vi "FGPA Area FWHM.vi"() -> ()   [LabVIEW 2017]
uses:
  <vilib>/rvi/interface/nirviOpenFPGA/nirviOpenFPGA.xnode
  <vilib>/rvi/interface/nirviCloseFPGA/nirviCloseFPGA.xnode
  <vilib>/rvi/Analysis/host/Public/NI_FpgaMspHost.lvlib
  <vilib>/rvi/interface/nirviMethod/nirviMethod.xnode
  <vilib>/rvi/errors/niLvFpgaMergeErrorWithErrorCode.vi
  <vilib>/FPGAPlugInAG/Dynamic/niLvFpga_Run_Dynamic.vi
  <vilib>/FPGAPlugInAG/Dynamic/niLvFpga_Reset_Dynamic.vi
  <vilib>/FPGAPlugInAG/Dynamic/niLvFpga_ConfigureFifo_Dynamic.vi
  <vilib>/FPGAPlugInAG/Dynamic/niLvFpga_ReadFifo_Dynamic.vi
  <vilib>/rvi/interface/nirviReadWriteControl/nirviReadWriteControl.xnode
  <extravilib>/ChannelInstances/Tag-bool.lvlib
  <vilib>/Analysis/NI_AALBase.lvlib
  FPGA Bitfiles/FPGAAreaFWHM_FPGATarget_ReadAnalog3Pulse_FqF0E97EYxI.lvbitx
  FADS_Area FWHM.vi
  <vilib>/Analysis/baseanly.llb/Mean (DBL).vi
  <vilib>/Utility/file.llb/Write Delimited Spreadsheet (DBL).vi
  <vilib>/rvi/Analysis/host/Private/Sample Rate To Loop Time (ticks).vi
  <vilib>/rvi/interface/Simulation/niFpgaSimulationCallBeginRW.vi
  <vilib>/rvi/errors/niLvFpgaAdjustHostInterfaceError.vi
  <vilib>/FPGAPlugInAG/Dynamic/niLvFpga_Close_Dynamic.vi
panel:
  out "Droplet Rate":dbl format="%0.2f"
  in  "Sample Name":string
  in  "Folder For Plots":path
  in  "Log Sorted Drop Data":bool
  in  "Tab Control":enum32{"Width", "FWHM"}(tab)
  in  "Min Width (us)":u32
  in  "Max Width (us)":u32=10000
  in  "Min FWHM (us)":i32
  in  "Max FWHM (us)":i32=10000
  out "Combined Histogram":T1(graph)
  out "Outside Sorted":cluster{"total":i32, "below":i32, "above":i32}
  out "Histogram Sorted Drops":T2(graph)
  out "Voltage Bins":i32
  out "Histogram":T2(graph)
  out "Outside Unsorted":cluster{"total":i32, "below":i32, "above":i32}
  out "Fraction Sorted":dbl
  out "Total Number of Droplets":i32
  out "Area Amplitude":i32[][](graph) caption="Area vs Amplitude"
  out "Area Bin Size":i32
  out "Voltage Bin Size":dbl=0.005
  in  "stop":bool
  out "FWHM Amplitude":i32[][](graph) caption="FWHM vs Amplitude"
  out "Buffer":u32
  out "Loop Time (ms)":u32
  out "Data Transfer":bool
  in  "Sort":bool
  out "Width Bin Size":i32
  in  "Save Plots":bool caption="Enable"
  out "Width Amplitude":i32[][](graph) caption="Width vs Amplitude"
  in  "Max Voltage (V)":dbl=10.0
  in  "Min Voltage (V)":dbl=10.0
  in  "Noise Level":dbl=0.2
  out "Sorted Droplets":u32
  in  "PMT Voltage":dbl(slide) scale=0.0..1.25
  in  "Add":bool
  in  "Reset":bool
  out "Voltage Trace":cluster{dbl[], dbl[]}[](graph)
  out "Sample Rate":dbl format="%#_6p"
  # "SORTING SETTINGS"
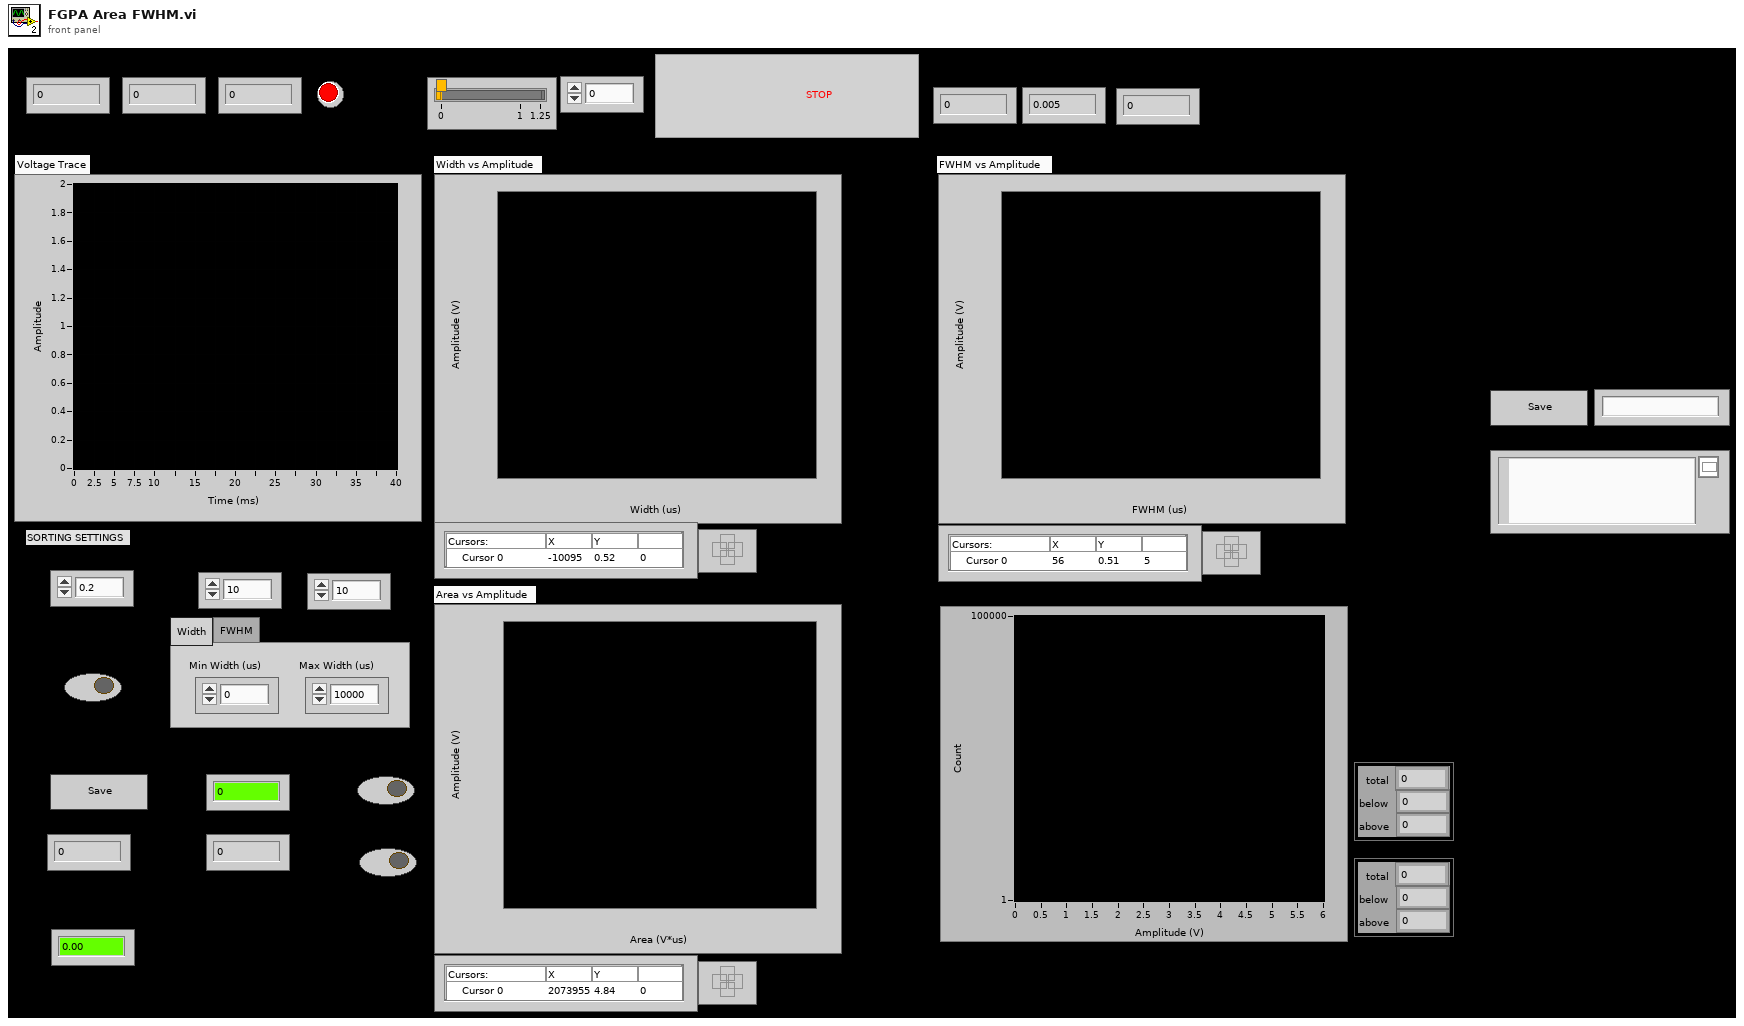
[diagram p1: front panel]
types:
  T1 = cluster{"X Values":dbl[], "Histogram: h(x)":i32[]}[]
  T2 = cluster{"X Values":dbl[], "Histogram: h(x)":i32[]}
  T3 = typedef "Tag-bool.lvlib/))Channel.ctl" = refnum<queue>
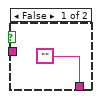
[diagram p3: hidden frame]
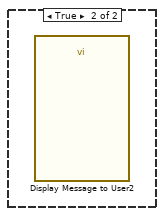
[diagram p4: hidden frame]
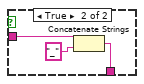
[diagram p6: hidden frame]
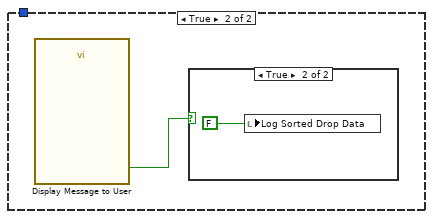
[diagram p7: hidden frame]
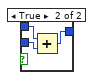
[diagram p9: hidden frame]
diagram:
  n1 = flat-sequence {
    tunnel: [w13] -> w5
    tunnel: [w12] -> w4
    tunnel: [w11] -> w3
    tunnel: [w10] -> w2
    tunnel: [w9] -> w1
    tunnel: [w47] -> w8
    tunnel: [w46] -> w7
    tunnel: [w45] -> w6
    tunnel: w5 -> [w44]
    tunnel: w4 -> [w43]
    tunnel: w3 -> [w42]
    tunnel: w2 -> [w39]
    tunnel: w1 -> [w41]
    tunnel: w8 -> [w317]
    tunnel: w7 -> [w316]
    tunnel: w6 -> [w315]
    frame #0 {
      w36 = 1000.0 ("x")
      w24 = 0.005 ("Voltage Bin Size")
      w11 = u32 100 ("milliseconds to wait")
      w32 = 0 ("element")
      # "Area Bin"
      # "INITIALIZE ARRAY WITH CORRECT BINS"
      # "Max Width Size"
      n2 = call-poly <vilib>:"Sample Rate To Loop Time.vi"("sample rate (S/s)"=200000.0 ("FPGA clock rate (Hz)"), "FPGA clock rate (Hz)"=40000000.0) -> ("actual sample rate (S/s)"=w38:dbl)  [unwired: 11 in, 2 out]
      "Sample Rate" <- w38
      n3 = Reciprocal(x=w38) -> (1/x=w9:dbl)
      n4 = Reciprocal(x=w38) -> (1/x=w20:dbl)
      n5 = Multiply(x=1000000.0, y=w20) -> (x*y=w19:dbl)
      n6 = Multiply(x=2.0, y=w19) -> (x*y=w14:dbl)
      n7 = To Long Integer(number=w14) -> (32bit integer=→"Width Bin Size":i32)
      n8 = Divide(x=10000.0 ("Max Width"), y=w14) -> (x/y=w22:dbl)
      n9 = Divide(x=11.0, y=w24) -> (x/y=w21:dbl)
      n10 = Divide(x=w38, y=1000.0) -> (x/y=w27:dbl)
      n11 = To Long Integer(number=w21) -> (32bit integer=w31:i32)
      "Voltage Bins" <- w31
      n12 = To Long Integer(number=w22) -> (32bit integer=w16:i32)
      n13 = Multiply(x=w11, y=w27) -> (x*y=w29:dbl)
      n14 = Initialize Array(w32, w16, w31) -> (w12:i32[][])
      n15 = To Unsigned Long Integer(number=w29) -> (unsigned 32bit integer=w10:u32)
      n16 = Divide(x=5000000.0, y=w36) -> (x/y=w35:dbl)
      n17 = To Long Integer(number=w35) -> (32bit integer=w34:i32)
      n18 = To Long Integer(number=w36) -> (32bit integer=→"Area Bin Size":i32)
      n19 = Initialize Array(w32, w34, w31) -> (w13:i32[][])
      "Voltage Bin Size" <- w24
    }
    frame #1 {
      w49 = u32 40000 ("Requested Depth")
      n20 = xnode "Open FPGA VI Reference"() -> ("FPGA VI Reference Out"=w69:refnum<k20>, "error out"=w65:errorcluster)  [unwired: 2 in]
      n21 = xnode "Invoke Method"("FPGA VI Reference In"=w69, "error in"=w65) -> ("FPGA VI Reference Out"=w66:refnum<k20>, "error out"=w64:errorcluster)
      n22 = xnode "Invoke Method"("FPGA VI Reference In"=w66, "error in"=w64, "Requested Depth"=w49) -> ("FPGA VI Reference Out"=w68:refnum<k20>, "error out"=w67:errorcluster)  [unwired: 1 out]
      n23 = xnode "Invoke Method"("FPGA VI Reference In"=w68, "Requested Depth"=w49) -> ("FPGA VI Reference Out"=w59:refnum<k20>)  [unwired: 1 in, 2 out]
      n24 = xnode "Invoke Method"("FPGA VI Reference In"=w59, "Requested Depth"=w49) -> ("FPGA VI Reference Out"=w50:refnum<k20>)  [unwired: 1 in, 2 out]
      n25 = xnode "Invoke Method"("FPGA VI Reference In"=w50, "error in"=w67) -> ("FPGA VI Reference Out"=w56:refnum<k20>, "error out"=w54:errorcluster)  [unwired: 1 in]
      n26 = Initialize Array(0.0 ("element"), 20 ("dimension size")) -> (w62:dbl[])
      n27 = for {
        N: w39 -> [_]
        tunnel: [w88] -> w57 mode=indexing
        tunnel: w41 -> [w87]
        i -> [w90]
        n28 = To Double Precision Float(number=w90) -> (double precision float=w89:dbl)
        n29 = Multiply(x=w87, y=w89) -> (x*y=w88:dbl)
      }
      n30 = Multiply(x=u32 2, y=w39) -> (x*y=w40:u32)
      n31 = Multiply(x=1000.0, y=w57) -> (x*y=w55:dbl[])
      n32 = while {
        tunnel: w56 -> [w86]
        tunnel: w55 -> [w72]
        tunnel: w42 -> [w82]
        tunnel: w40 -> [w84]
        tunnel: w54 -> [w81]
        tunnel: [w80] -> w45
        tunnel: [w76] -> w53
        stop <- w77 stop-if-true
        # "Data Stean of Voltage Trace"
        n33 = Wait (ms)(milliseconds to wait=w82) -> ()  [unwired: 1 out]
        n34 = xnode "Invoke Method"("FPGA VI Reference In"=w86, "error in"=w81, "Number of Elements"=w84, "Timeout (ms)"=5000) -> ("error out"=w80:errorcluster, "Data"=w85:void[])  [unwired: 2 out]
        n35 = call "Conversion_to_Volt.vi"("Data"=w85) -> ("Array"=w71:dbl[])  [unwired: 10 in]
        n36 = Decimate 1D Array(w71) -> (w75:dbl[], w73:dbl[])
        n37 = Bundle(w72, w75) -> ()  [unwired: 1 in, 1 out]
        n38 = Bundle(w72, w73) -> (w70:cluster{dbl[], dbl[]})  [unwired: 1 in]
        n39 = Build Array(w70) -> (→"Voltage Trace":cluster{dbl[], dbl[]}[])
        n40 = Unbundle By Name(w80) -> ("status"=w79:bool)
        n41 = Or(x=w79, y="stop") -> (x .or. y?=w77:bool)
        n42 = call <extravilib>:"Write.vi"("element"=w77) -> ("channel"=w76:T3)  [unwired: 1 out]
      }
      n43 = while {
        shift-right: [w200] -> w46
        shift-left: w54 -> [w225]
        shift-right: [w156] -> w47
        shift-left: w56 -> [w228]
        shift-right: [w220] -> _
        shift-left: w62 -> [w221]
        shift-right: [w213] -> _
        shift-left: 0 ("dimension size") -> [w214]
        shift-right: [w178] -> _
        shift-left: u32 0 ("millisecond timer value") -> [w179]
        tunnel: w43 -> [w170]
        tunnel: w53 -> [w162]
        tunnel: w44 -> [w148]
        shift-right: [w135] -> _
        shift-left: 0 -> [w138]
        stop <- w224 stop-if-true
        w116 = 0.0 ("min")
        w115 = 11.0 ("max")
        w150 = u32 4
        w175 = u32 4 ("y")
        # "Collected Drops"
        # "To Waste Drops"
        # "All Drops"
        # "PLOT FILTERED CUMULATED 1D HISTOGRAM OF PEAK AMPLITUDE"
        # "Area"
        # "FWHM"
        # "Width"
        # "FWHM"
        # "Area"
        # "Amplitude"
        # "Width"
        # "Check for Data Transfer Slippage"
        # "Amplitude"
        # "NUMBER OF SAMPLES MULTIPLE OF FOUR"
        # "Write to FPGA Controls and Read from FPGA Indicators"
        n44 = local read "Reset"() -> (w192:bool)
        n45 = Wait (ms)(milliseconds to wait=u32 100) -> ()  [unwired: 1 out]
        n46 = call "Conversion.vi"("Sorting Threshold"="Max Voltage (V)") -> ("Numeric 2"=w189:i16)  [unwired: 9 in, 1 out]
        n47 = call "Conversion.vi"("Sorting Threshold"="Noise Level") -> ("Numeric 2"=w206:i16)  [unwired: 9 in, 1 out]
        n48 = call "Conversion.vi"("Sorting Threshold"="PMT Voltage") -> ("Numeric 2"=w212:i16)  [unwired: 9 in, 1 out]
        n49 = call "Conversion.vi"("Sorting Threshold"="Min Voltage (V)") -> ("Numeric 2"=w188:i16)  [unwired: 9 in, 1 out]
        n50 = Equal?(x="Tab Control", y=enum32{"Width", "FWHM"}."FWHM") -> (x = y?=w104:bool)
        n51 = Tick Count (ms)() -> (millisecond timer value=w178:u32)
        n52 = Equal?(x=20, y=w214) -> (x = y?=w216:bool)
        n53 = Subtract(x=w178, y=w179) -> (x-y=→"Loop Time (ms)":u32)
        n54 = xnode "Read/Write Control"("FPGA VI Reference In"=w228, "error in"=w225, "PMT Voltage"=w212, "Noise Level"=w206, "Min Sorting Threshold"=w188, "Max Sorting Threshold"=w189, "Min Width"="Min Width (us)", "Max Width"="Max Width (us)", "Count Reset"=w192, "Sort"="Sort", "Trigger Length"=u32 50, "Min FWHM"="Min FWHM (us)", "Max FWHM"="Max FWHM (us)", "FWHM"=w104) -> ("FPGA VI Reference Out"=w227:refnum<k20>, "error out"=w226:errorcluster, "Event Count"=→"Sorted Droplets")
        n55 = Increment(x=w214) -> (x+1=w215:i32)
        n56 = Select(t=0, s=w216, f=w215) -> (s? t:f=w213:i32)
        n57 = xnode "Invoke Method"("FPGA VI Reference In"=w227, "error in"=w226, "Number of Elements"=u32 0, "Timeout (ms)"=-1) -> ("FPGA VI Reference Out"=w210:refnum<k20>, "error out"=w201:errorcluster, "Elements Remaining"=w176)  [unwired: 1 out]
        "Buffer" <- w176
        n58 = Quotient & Remainder(x=w176, y=w175) -> (floor(x/y)=w174:u32)  [unwired: 1 out]
        n59 = Multiply(x=w174, y=w175) -> (x*y=w173:u32)
        n60 = xnode "Invoke Method"("FPGA VI Reference In"=w210, "error in"=w201, "Number of Elements"=w173, "Timeout (ms)"=-1) -> ("FPGA VI Reference Out"=w184:refnum<k20>, "error out"=w200:errorcluster, "Data"=w125:void[])  [unwired: 1 out]
        n61 = xnode "Invoke Method"("FPGA VI Reference In"=w184, "Number of Elements"=u32 0, "Timeout (ms)"=-1) -> ("FPGA VI Reference Out"=w157:refnum<k20>, "Elements Remaining"=w152)  [unwired: 1 in, 2 out]
        n62 = Quotient & Remainder(x=w152, y=w150) -> (floor(x/y)=w149:u32)  [unwired: 1 out]
        n63 = Multiply(x=w149, y=w150) -> (x*y=w151:u32)
        n64 = local read "Folder For Plots"() -> (w91:path)
        n65 = xnode "Invoke Method"("FPGA VI Reference In"=w157, "Number of Elements"=w151, "Timeout (ms)"=-1) -> ("FPGA VI Reference Out"=w156:refnum<k20>, "Data"=w124:void[])  [unwired: 1 in, 2 out]
        n66 = local read "Add"() -> (w95:bool)
        n67 = And(x=w95, y="Log Sorted Drop Data") -> (x .and. y?=w94:bool)
        n68 = Insert Into Array(array=w124, new element=w125) -> (w141:void[])  [unwired: 1 in]
        n69 = Decimate 1D Array(w125) -> (w121:void[])  [unwired: 3 out]
        n70 = Decimate 1D Array(w124) -> (w101:void[], w122:void[], w99:void[], w100:void[])
        n71 = Decimate 1D Array(w141) -> (w140:void[], w185:void[], w108:void[], w168:void[])
        n72 = To Word Integer(number=w121) -> (16bit integer=w126:i16[])
        n73 = local read "Loop Time (ms)"() -> (w197:u32)
        n74 = To Word Integer(number=w122) -> (16bit integer=w123:i16[])
        n75 = Absolute Value(x=w108) -> (abs(x)=w107:dbl[])
        n76 = call "Conversion_to_Volt.vi"("Data"=w126) -> ("Array"=w120:dbl[])  [unwired: 10 in]
        n77 = call "Conversion_to_Volt.vi"("Data"=w123) -> ("Array"=w102:dbl[])  [unwired: 10 in]
        n78 = case shown="True" w94 {
          tunnel: w102 -> [_ w290]
          tunnel: w101 -> [_ w289]
          tunnel: w100 -> [_ w288]
          tunnel: w99 -> [_ w287]
          tunnel: w91 -> [_ w283]
          frame False {
          }
          frame True {
            n79 = Multiply(x=w289, y=-1) -> (x*y=w286:i32)
            n80 = Absolute Value(x=w287) -> (abs(x)=w284:dbl[])
            n81 = Equal?(x=w283, y=path "") -> (x = y?=w281:bool)
            n82 = case shown="False" w281 {
              tunnel: w290 -> [w304 _]
              tunnel: w288 -> [w303 _]
              tunnel: w286 -> [w302 _]
              tunnel: w284 -> [w301 _]
              tunnel: w283 -> [w293 _]
              frame False {
                w299 = TRUE ("append to file? (new file:F)")
                n83 = local read "Sample Name"() -> (w291:string)
                n84 = Build Array(w302, w303, w301, w304) -> (w300:dbl[])
                n85 = Not Equal?(x="", y=w291) -> (x != y?=w296:bool)
                n86 = case shown="False" w296 {
                  tunnel: w291 -> [_ w307]
                  tunnel: ["Sample" ("WidthVsAmplitude") w306] -> w294
                  frame False {
                  }
                  frame True {
                    n87 = Concatenate Strings(w307, "_") -> (w306:string)
                  }
                }
                n88 = Concatenate Strings(w294, "SortedDropProperties.txt" ("WidthVsAmplitude")) -> (w297:string)
                n89 = Build Path(base path=w293, name or relative path=w297) -> (appended path=w292:path)
                n90 = call-poly <vilib>:"Write Delimited Spreadsheet.vi"("file path (dialog if empty)"=w292, "2D data"=w300, "append to file? (new file:F)"=w299, "transpose? (no:F)"=w299) -> ()  [unwired: 10 in, 2 out]
              }
              frame True {
                n91 = call "Display Message to User"() -> ("OK"=w309:bool)  [unwired: 10 in, 1 out]
                n92 = case shown="True" w309 {
                  frame False {
                  }
                  frame True {
                    n93 = local write "Log Sorted Drop Data"(FALSE) -> ()
                  }
                }
              }
            }
          }
        }
        n94 = Greater?(x=0 ("y"), y=w140) -> (0:w181:bool)
        n95 = To Double Precision Float(number=w197) -> (double precision float=w198:dbl)
        n96 = Multiply(x=w140, y=-1) -> (x*y=w165:i32)
        n97 = Divide(x=w198, y=1000.0) -> (x/y=w196:dbl)
        n98 = And Array Elements(Boolean array=w181) -> (logical AND=→"Data Transfer":bool)
        n99 = Array Size(array=w140) -> (size(s)=w131:i32)
        n100 = To Double Precision Float(number=w131) -> (double precision float=w195:dbl)
        n101 = Divide(x=w195, y=w196) -> (x/y=w222:dbl)
        n102 = Replace Array Subset(array=w221, new element=w222, index=w214) -> (w220:dbl[])
        n103 = local read "Add"() -> (w132:bool)
        n104 = call-poly <vilib>:"Mean.vi"("X"=w220) -> ("mean"=→"Droplet Rate":dbl)  [unwired: 1 out]
        n105 = case shown="False" w132 {
          tunnel: w138 -> [w311 w314]
          tunnel: w131 -> [_ w313]
          tunnel: [w311 w312] -> w134
          frame False {
          }
          frame True {
            n106 = Add(x=w314, y=w313) -> (x+y=w312:i32)
          }
        }
        "Total Number of Droplets" <- w134
        n107 = local read "Sorted Droplets"() -> (w137:u32)
        n108 = local read "Reset"() -> (w133:bool)
        n109 = To Word Integer(number=w185) -> (16bit integer=w186:i16[])
        n110 = call "Conversion_to_Volt.vi"("Data"=w186) -> ("Array"=w127:dbl[])  [unwired: 10 in]
        n111 = Divide(x=w137, y=w134) -> (x/y=→"Fraction Sorted":dbl)
        n112 = local read "Voltage Bin Size"() -> (w142:dbl)
        n113 = local read "Width Bin Size"() -> (w166:i32)
        n114 = local read "Width Bin Size"() -> (w169:i32)
        n115 = Select(t=w131, s=w133, f=w134) -> (s? t:f=w135:i32)
        n116 = local read "Area Bin Size"() -> (w145:i32)
        n117 = Quotient & Remainder(x=w168, y=w169) -> (floor(x/y)=w167:i32)  [unwired: 1 out]
        n118 = Quotient & Remainder(x=w107, y=w145) -> (floor(x/y)=w146:dbl[])  [unwired: 1 out]
        n119 = Quotient & Remainder(x=w127, y=w142) -> (floor(x/y)=w194:dbl[])  [unwired: 1 out]
        n120 = Quotient & Remainder(x=w165, y=w166) -> (floor(x/y)=w164:i32)  [unwired: 1 out]
        n121 = To Long Integer(number=w194) -> (32bit integer=w147:i32[])
        n122 = local read "Histogram Sorted Drops"() -> (w118:T2)
        n123 = local read "Histogram"() -> (w129:T2)
        n124 = local read "Outside Unsorted"() -> (w128:cluster{"total":i32, "below":i32, "above":i32})
        n125 = local read "Outside Sorted"() -> (w117:cluster{"total":i32, "below":i32, "above":i32})
        n126 = call "2DHisto.vi"("Array 2"=w147, "Array 4"=w164, "Array"=w170) -> ("Array 3"=w172:i32[][])  [unwired: 8 in]
        n127 = call "2DHisto.vi"("Array 2"=w147, "Array 4"=w167, "Array"=w170) -> ("Array 3"=w160:i32[][])  [unwired: 8 in]
        n128 = call "2DHisto.vi"("Array 2"=w147, "Array 4"=w146, "Array"=w148) -> ("Array 3"=w144:i32[][])  [unwired: 8 in]
        n129 = local read "Voltage Bins"() -> (w114:i32)
        n130 = local read "Width Amplitude"() -> (w193:i32[][])
        n131 = local read "Area Amplitude"() -> (w143:i32[][])
        n132 = local read "FWHM Amplitude"() -> (w158:i32[][])
        n133 = call "HistoPlotter.vi"("Filtered Histogram"=w129, "Add in"="Add", "Reset in"="Reset", "Outside"=w128, "Array"=w120, "min"=w116, "max"=w115, "Voltage Bins"=w114) -> ("Histogram Graph"=w97:T2, "# outside"=→"Outside Unsorted":cluster{"total":i32, "below":i32, "above":i32})  [unwired: 6 in]
        "Histogram" <- w97
        n134 = call "HistoPlotter.vi"("Filtered Histogram"=w118, "Add in"="Add", "Reset in"="Reset", "Outside"=w117, "Array"=w102, "min"=w116, "max"=w115, "Voltage Bins"=w114) -> ("Histogram Graph"=w92:T2, "# outside"=→"Outside Sorted":cluster{"total":i32, "below":i32, "above":i32})  [unwired: 6 in]
        "Histogram Sorted Drops" <- w92
        n135 = call "2DPlotter.vi"("Reset"="Reset", "Add"="Add", "New Data"=w160, "Plot In"=w158) -> ("Plot Out"=w159:i32[][])  [unwired: 7 in]
        "FWHM Amplitude" <- w159
        n136 = call "2DPlotter.vi"("Reset"="Reset", "Add"="Add", "New Data"=w144, "Plot In"=w143) -> ("Plot Out"=w139:i32[][])  [unwired: 7 in]
        "Area Amplitude" <- w139
        n137 = call "2DPlotter.vi"("Reset"="Reset", "Add"="Add", "New Data"=w172, "Plot In"=w193) -> ("Plot Out"=w183:i32[][])  [unwired: 7 in]
        "Width Amplitude" <- w183
        n138 = Build Array(w92, w97) -> (→"Combined Histogram":T1)
        n139 = case shown="True" "Save Plots" {
          tunnel: w183 -> [_ w237]
          tunnel: w159 -> [_ w236]
          tunnel: w139 -> [_ w235]
          tunnel: "Folder For Plots" -> [_ w234]
          tunnel: w97 -> [_ w233]
          tunnel: "Save Plots" -> [_ w232]
          tunnel: w92 -> [_ w229]
          frame False {
          }
          frame True {
            n140 = Equal?(x=w234, y=path "") -> (x = y?=w231:bool)
            n141 = case shown="False" w231 {
              tunnel: w237 -> [w275 _]
              tunnel: w236 -> [w273 _]
              tunnel: w235 -> [w271 _]
              tunnel: w234 -> [w253 _]
              tunnel: w233 -> [w263 _]
              tunnel: w232 -> [w238 _]
              tunnel: w229 -> [w254 _]
              frame False {
                n142 = Unbundle(w263) -> ("X Values"=w262:dbl[], "Histogram: h(x)"=w261:i32[])
                n143 = Unbundle(w254) -> ("X Values"=w256:dbl[], "Histogram: h(x)"=w255:i32[])
                n144 = Not Equal?(x="", y="Sample Name") -> (x != y?=w250:bool)
                n145 = case shown="True" w250 {
                  tunnel: "Sample Name" -> [_ w279]
                  tunnel: ["" w278] -> w247
                  frame False {
                  }
                  frame True {
                    n146 = Concatenate Strings(w279, "_") -> (w278:string)
                  }
                }
                n147 = call "Convert to Dynamic Data2"("2D Array"=w271) -> ("Dynamic Data Type"=w272:dynamicdata)  [unwired: 3 in]
                n148 = call "Convert to Dynamic Data3"("2D Array"=w275) -> ("Dynamic Data Type"=w276:dynamicdata)  [unwired: 3 in]
                n149 = call "Convert to Dynamic Data"("2D Array"=w273) -> ("Dynamic Data Type"=w274:dynamicdata)  [unwired: 3 in]
                n150 = call "Convert to Dynamic Data5"("Array"=w261) -> ("Dynamic Data Type"=w268:dynamicdata)  [unwired: 3 in]
                n151 = call "Convert to Dynamic Data4"("Array"=w262) -> ("Dynamic Data Type"=w270:dynamicdata)  [unwired: 3 in]
                n152 = call "Convert to Dynamic Data7"("Array"=w255) -> ("Dynamic Data Type"=w258:dynamicdata)  [unwired: 3 in]
                n153 = call "Convert to Dynamic Data6"("Array"=w256) -> ("Dynamic Data Type"=w260:dynamicdata)  [unwired: 3 in]
                n154 = Concatenate Strings(w247, "WidthAmplitude" ("WidthVsAmplitude")) -> (w251:string)
                n155 = Concatenate Strings(w247, "FWHMAmplitude" ("WidthVsAmplitude")) -> (w243:string)
                n156 = Concatenate Strings(w247, "AreaAmplitude" ("WidthVsAmplitude")) -> (w245:string)
                n157 = Concatenate Strings(w247, "HistogramUnsorted.txt" ("WidthVsAmplitude")) -> (w241:string)
                n158 = Concatenate Strings(w247, "HistogramSorted.txt" ("WidthVsAmplitude")) -> (w239:string)
                n159 = Merge Signals(w270, w268) -> (w269:dynamicdata)
                n160 = Merge Signals(w260, w258) -> (w259:dynamicdata)
                n161 = Build Path(base path=w253, name or relative path=w251) -> (appended path=w267:path)
                n162 = Build Path(base path=w253, name or relative path=w243) -> (appended path=w264:path)
                n163 = Build Path(base path=w253, name or relative path=w245) -> (appended path=w265:path)
                n164 = Build Path(base path=w253, name or relative path=w241) -> (appended path=w266:path)
                n165 = Build Path(base path=w253, name or relative path=w239) -> (appended path=w257:path)
                n166 = call "Write To Measurement File2"("Signals"=w276, "Enable"=w238, "new_file"=w238, "Filename"=w267) -> ()  [unwired: 13 in, 3 out]
                n167 = call "Write To Measurement File"("Signals"=w274, "Enable"=w238, "new_file"=w238, "Filename"=w264) -> ()  [unwired: 13 in, 3 out]
                n168 = call "Write To Measurement File3"("Signals"=w272, "Enable"=w238, "new_file"=w238, "Filename"=w265) -> ()  [unwired: 13 in, 3 out]
                n169 = call "Write To Measurement File4"("Signals"=w269, "Enable"=w238, "new_file"=w238, "Filename"=w266) -> ()  [unwired: 13 in, 3 out]
                n170 = call "Write To Measurement File5"("Signals"=w259, "Enable"=w238, "new_file"=w238, "Filename"=w257) -> ()  [unwired: 13 in, 3 out]
              }
              frame True {
                n171 = call "Display Message to User2"() -> ()  [unwired: 10 in, 2 out]
              }
            }
          }
        }
        n172 = Unbundle By Name(w200) -> ("status"=w171:bool)
        n173 = call <extravilib>:"Read.vi"("channel"=w162) -> ("element"=w161:bool)  [unwired: 1 in, 1 out]
        n174 = Or(x=w171, y=w161) -> (x .or. y?=w224:bool)
      }
    }
    frame #2 {
      n175 = Merge Errors(w315, w316) -> (w318:errorcluster)
      n176 = xnode "Close FPGA VI Reference"("FPGA VI Reference In"=w317, "error in"=w318) -> ("error out"=w319:errorcluster)
      n177 = call <vilib>:"Simple Error Handler.vi"("error in (no error)"=w319) -> ()  [unwired: 4 in, 5 out]
    }
  }
